vi "FPGA_EncoderReadOutput.vi"(8 "error in (no error)":errorcluster, 11 "EncoderDevRef":T1) -> (0 "error out":errorcluster, 1 "Direction":bool, 2 "Value":i32, 3 "EncoderDevRef":T1)   [LabVIEW 2017]
uses:
  <vilib>/Rock Robotics/SystemInterfaces/Encoder/FPGA_EncoderDevRef.ctl
  <vilib>/Rock Robotics/SystemInterfaces/Encoder/FPGA_EncoderIdx.ctl
  <vilib>/Rock Robotics/SystemInterfaces/System/FPGA_SystemFPGA Ref Global.vi
  <vilib>/Utility/error.llb/Error Cluster From Error Code.vi
  <vilib>/rvi/errors/niLvFpgaAdjustHostInterfaceError.vi
  <vilib>/rvi/interface/nirviReadWriteControl/nirviReadWriteControl.xnode
  <vilib>/Rock Robotics/SystemInterfaces/System/FPGA_SystemFRC FPGA Ref.ctl
  NiFpgaLv.dll
  <vilib>/rvi/interface/Simulation/niFpgaSimulationCallBeginRW.vi
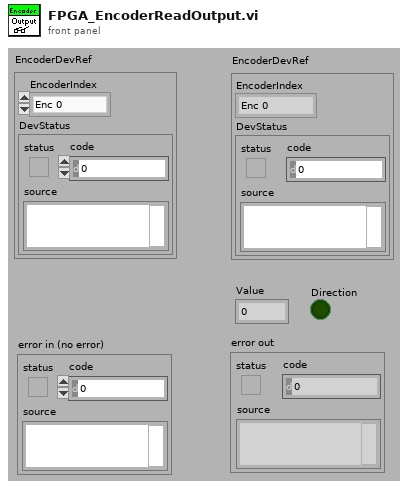
[diagram p1: front panel]
types:
  T1 = typedef "FPGA_EncoderDevRef.ctl" = cluster{"EncoderIndex":T2, "DevStatus":errorcluster}
  T2 = typedef "FPGA_EncoderIdx.ctl" = enum8{"Enc 0", "Enc 1", "Enc 2", "Enc 3", "Enc 4", "Enc 5", "Enc 6", "Enc 7", "Invalid"}
  T3 = typedef "FPGA_SystemFRC FPGA Ref.ctl" = refnum<k20>
  T4 = cluster{"Direction":bool, "Value":fxp<+/-,31,31>}
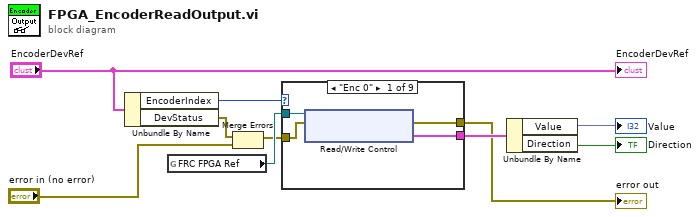
[diagram p0: block diagram]
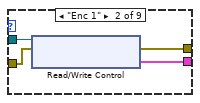
[diagram p2: hidden frame]
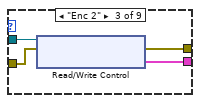
[diagram p3: hidden frame]
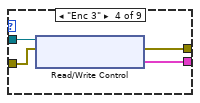
[diagram p4: hidden frame]
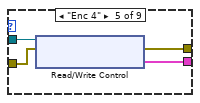
[diagram p5: hidden frame]
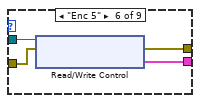
[diagram p6: hidden frame]
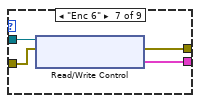
[diagram p7: hidden frame]
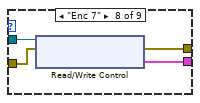
[diagram p8: hidden frame]
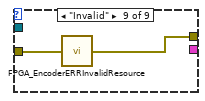
[diagram p9: hidden frame]
diagram:
  n1 = Unbundle By Name("EncoderDevRef") -> ("EncoderIndex"=w5:T2, "DevStatus"=w2:errorcluster)
  n2 = global read "FPGA_SystemFPGA Ref Global.vi" "FRC FPGA Ref"() -> (w4:T3)
  n3 = Merge Errors(w2, "error in (no error)") -> (w3:errorcluster)
  n4 = case shown="\"Enc 0\"" w5 {
    tunnel: w4 -> [w11 w15 w19 w23 w27 w31 w35 w39 _]
    tunnel: w3 -> [w12 w16 w20 w24 w28 w32 w36 w40 w44]
    tunnel: [w13 w17 w21 w25 w29 w33 w37 w41 w43] -> w8
    tunnel: [w14 w18 w22 w26 w30 w34 w38 w42 _] -> w10
    frame "Enc 0" {
      n5 = xnode "Read/Write Control"("FPGA VI Reference In"=w11, "error in"=w12) -> ("error out"=w13:errorcluster, "Encoder0.Output"=w14:T4)  [unwired: 1 out]
    }
    frame "Enc 1" {
      n6 = xnode "Read/Write Control"("FPGA VI Reference In"=w15, "error in"=w16) -> ("error out"=w17:errorcluster, "Encoder1.Output"=w18:T4)  [unwired: 1 out]
    }
    frame "Enc 2" {
      n7 = xnode "Read/Write Control"("FPGA VI Reference In"=w19, "error in"=w20) -> ("error out"=w21:errorcluster, "Encoder2.Output"=w22:T4)  [unwired: 1 out]
    }
    frame "Enc 3" {
      n8 = xnode "Read/Write Control"("FPGA VI Reference In"=w23, "error in"=w24) -> ("error out"=w25:errorcluster, "Encoder3.Output"=w26:T4)  [unwired: 1 out]
    }
    frame "Enc 4" {
      n9 = xnode "Read/Write Control"("FPGA VI Reference In"=w27, "error in"=w28) -> ("error out"=w29:errorcluster, "Encoder4.Output"=w30:T4)  [unwired: 1 out]
    }
    frame "Enc 5" {
      n10 = xnode "Read/Write Control"("FPGA VI Reference In"=w31, "error in"=w32) -> ("error out"=w33:errorcluster, "Encoder5.Output"=w34:T4)  [unwired: 1 out]
    }
    frame "Enc 6" {
      n11 = xnode "Read/Write Control"("FPGA VI Reference In"=w35, "error in"=w36) -> ("error out"=w37:errorcluster, "Encoder6.Output"=w38:T4)  [unwired: 1 out]
    }
    frame "Enc 7" {
      n12 = xnode "Read/Write Control"("FPGA VI Reference In"=w39, "error in"=w40) -> ("error out"=w41:errorcluster, "Encoder7.Output"=w42:T4)  [unwired: 1 out]
    }
    frame "Invalid" {
      n13 = call <vilib>:"FPGA_EncoderERRInvalidResource.vi"("error in (no error)"=w44) -> ("error out"=w43:errorcluster)
    }
  }
  "error out" <- w8
  n14 = Unbundle By Name(w10) -> ("Value"=→"Value":fxp<+/-,31,31>, "Direction"=→"Direction":bool)
  "EncoderDevRef" <- "EncoderDevRef"
